vi "setServerUrl.vi"(8 "error in (no error)":errorcluster, 10 "serverUrl":string, 11 "repoHandler in":refnum<class "repoHandler.lvclass">) -> (0 "error out":errorcluster, 3 "repoHandler out":refnum<class "repoHandler.lvclass">)   [LabVIEW 2013, in "repoHandler.lvclass"]
uses:
  repoHandler.lvclass
  repoHandler.lvclass/repoHandler.ctl
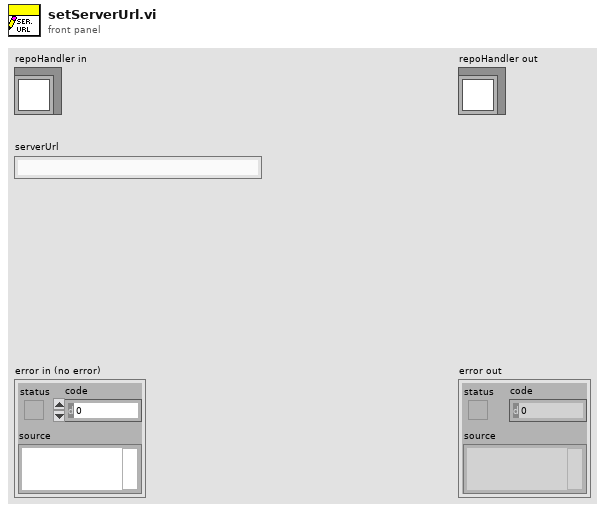
[diagram p1: front panel]
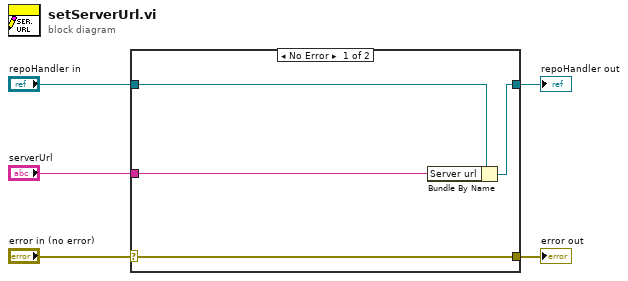
[diagram p0: block diagram]
diagram:
  n1 = case shown="No Error" "error in (no error)" {
    selector: "error in (no error)" -> [w9 w10]
    tunnel: [w9 w10] -> w4
    tunnel: [w7 w11] -> w2
    tunnel: "repoHandler in" -> [w8 w11]
    tunnel: "serverUrl" -> [w6 _]
    frame No Error {
      n2 = Bundle By Name(cluster=w8, "Server url"=w6) -> (w7:refnum<class "repoHandler.lvclass">)
    }
    frame Error {
    }
  }
  "error out" <- w4
  "repoHandler out" <- w2
